vi "Sort Array__ogtk.vi"   [LabVIEW 2014]
doc: "This polymorphic VI sorts 1D or 2D arrays. You can specify whether to sort in ascending or descending order. For 2D arrays, you can specify whether to sort by column or row and which column or row to sort by."
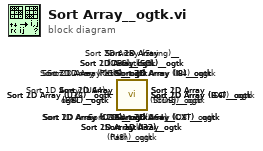
[diagram p0: block diagram]
diagram:
  n1 = call <userlib>:"Sort 2D Array (U64)__ogtk.vi"() -> ()  [unwired: 8 in, 4 out]
  n2 = call <userlib>:"Sort 2D Array (I64)__ogtk.vi"() -> ()  [unwired: 8 in, 4 out]
  n3 = call <userlib>:"Sort 1D Array (U64)__ogtk.vi"() -> ()  [unwired: 10 in, 2 out]
  n4 = call <userlib>:"Sort 1D Array (I64)__ogtk.vi"() -> ()  [unwired: 10 in, 2 out]
  n5 = call <userlib>:"Sort 2D Array (String)__ogtk.vi"() -> ()  [unwired: 8 in, 4 out]
  n6 = call <userlib>:"Sort 2D Array (Path)__ogtk.vi"() -> ()  [unwired: 8 in, 4 out]
  n7 = call <userlib>:"Sort 1D Array (String)__ogtk.vi"() -> ()  [unwired: 10 in, 2 out]
  n8 = call <userlib>:"Sort 1D Array (Path)__ogtk.vi"() -> ()  [unwired: 10 in, 2 out]
  n9 = call <userlib>:"Sort 2D Array (U8)__ogtk.vi"() -> ()  [unwired: 8 in, 4 out]
  n10 = call <userlib>:"Sort 2D Array (U32)__ogtk.vi"() -> ()  [unwired: 8 in, 4 out]
  n11 = call <userlib>:"Sort 2D Array (U16)__ogtk.vi"() -> ()  [unwired: 8 in, 4 out]
  n12 = call <userlib>:"Sort 2D Array (SGL)__ogtk.vi"() -> ()  [unwired: 8 in, 4 out]
  n13 = call <userlib>:"Sort 2D Array (I8)__ogtk.vi"() -> ()  [unwired: 8 in, 4 out]
  n14 = call <userlib>:"Sort 2D Array (I32)__ogtk.vi"() -> ()  [unwired: 8 in, 4 out]
  n15 = call <userlib>:"Sort 2D Array (I16)__ogtk.vi"() -> ()  [unwired: 8 in, 4 out]
  n16 = call <userlib>:"Sort 2D Array (EXT)__ogtk.vi"() -> ()  [unwired: 8 in, 4 out]
  n17 = call <userlib>:"Sort 2D Array (DBL)__ogtk.vi"() -> ()  [unwired: 8 in, 4 out]
  n18 = call <userlib>:"Sort 2D Array (CSG)__ogtk.vi"() -> ()  [unwired: 8 in, 4 out]
  n19 = call <userlib>:"Sort 2D Array (CXT)__ogtk.vi"() -> ()  [unwired: 8 in, 4 out]
  n20 = call <userlib>:"Sort 2D Array (CDB)__ogtk.vi"() -> ()  [unwired: 8 in, 4 out]
  n21 = call <userlib>:"Sort 1D Array (U8)__ogtk.vi"() -> ()  [unwired: 10 in, 2 out]
  n22 = call <userlib>:"Sort 1D Array (U32)__ogtk.vi"() -> ()  [unwired: 10 in, 2 out]
  n23 = call <userlib>:"Sort 1D Array (U16)__ogtk.vi"() -> ()  [unwired: 10 in, 2 out]
  n24 = call <userlib>:"Sort 1D Array (SGL)__ogtk.vi"() -> ()  [unwired: 10 in, 2 out]
  n25 = call <userlib>:"Sort 1D Array (I8)__ogtk.vi"() -> ()  [unwired: 10 in, 2 out]
  n26 = call <userlib>:"Sort 1D Array (I32)__ogtk.vi"() -> ()  [unwired: 10 in, 2 out]
  n27 = call <userlib>:"Sort 1D Array (I16)__ogtk.vi"() -> ()  [unwired: 10 in, 2 out]
  n28 = call <userlib>:"Sort 1D Array (EXT)__ogtk.vi"() -> ()  [unwired: 10 in, 2 out]
  n29 = call <userlib>:"Sort 1D Array (DBL)__ogtk.vi"() -> ()  [unwired: 10 in, 2 out]
  n30 = call <userlib>:"Sort 1D Array (CSG)__ogtk.vi"() -> ()  [unwired: 10 in, 2 out]
  n31 = call <userlib>:"Sort 1D Array (CXT)__ogtk.vi"() -> ()  [unwired: 10 in, 2 out]
  n32 = call <userlib>:"Sort 1D Array (CDB)__ogtk.vi"() -> ()  [unwired: 10 in, 2 out]
